vi "DUAL GAUGE-Test ADC.vi"(8 "Fehler (Eingang)":errorcluster, 11 "Referenz in":refnum<visa-resource-name>) -> (0 "Cluster (Ausgang)":errorcluster, 1 "ADC Channel 3":dbl format="%.4f", 2 "ADC Channel 2":dbl format="%.4f", 3 "Referenz out":refnum<visa-resource-name>, 4 "ADC Channel 4":dbl format="%.4f", 5 "ADC Channel 1":dbl format="%.4f")   [LabVIEW 2013, in "Dual Gauge.lvlib"]
uses:
  Dual Gauge.lvlib
panel:
  # "V"
  # "V"
  # "V"
  # "V"
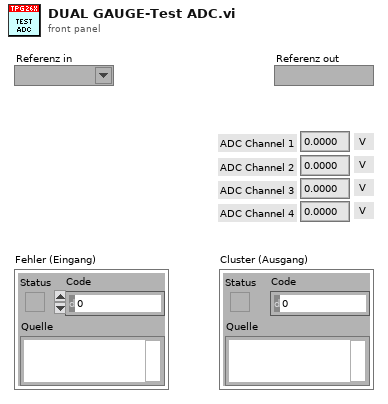
[diagram p1: front panel]
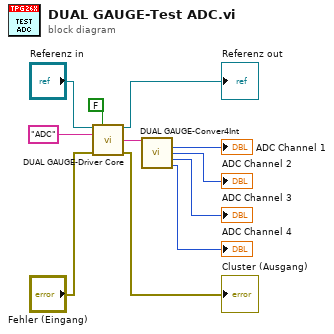
[diagram p0: block diagram]
diagram:
  n1 = call "DUAL GAUGE-Driver Core.vi"("Referenz in"="Referenz in", "Write/Read"=FALSE, "Command"="ADC", "Fehler (Eingang)"="Fehler (Eingang)") -> ("Referenz out"=→"Referenz out":refnum<visa-resource-name>, "String Out"=w6:string, "Cluster (Ausgang)"=→"Cluster (Ausgang)":errorcluster)  [unwired: 9 in]
  n2 = call "DUAL GAUGE-Conver4Int.vi"("String in"=w6) -> ("ADC CH 1 out"=→"ADC Channel 1":u16, "Integer2 out"=→"ADC Channel 2":u16, "Integer3 out"=→"ADC Channel 3":u16, "Integer4 out"=→"ADC Channel 4":u16)  [unwired: 11 in]
